vi "Get All Logging Properties.vi"(8 "error in":errorcluster, 11 "logging ref":T3=18446744073709551615 format="%.0x") -> (0 "error out":errorcluster, 1 "log thresholds":T2 {"Segment Files By" items=["Time", "Size"]}, 2 "log file info":T1, 3 "logging ref out":T3 format="%.0x")   [LabVIEW 2020, in "AIM ARINC 664 Scripting.lvlib"]
uses:
  AIM ARINC 664 Scripting.lvlib
  <vilib>/NI VeriStand/Custom Device API/Custom Device Item Ref.ctl
  Shared/loggingThreshold_types.ctl
  Shared/logFileInfo_types.ctl
  <vilib>/NI VeriStand/Custom Device API/Custom Device API.lvlib
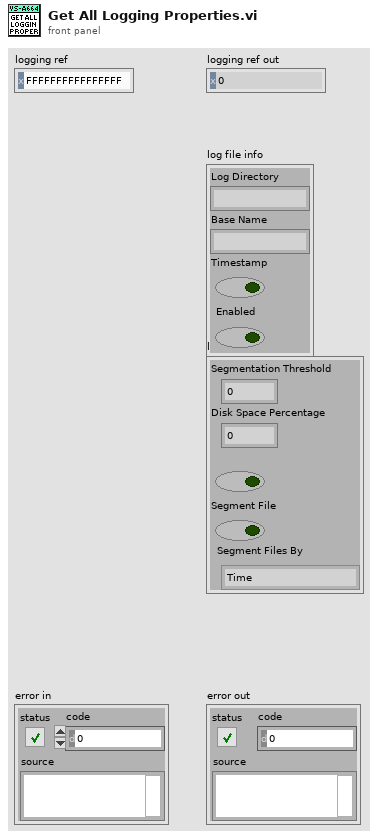
[diagram p1: front panel]
types:
  T1 = typedef "logFileInfo_types.ctl" = cluster{"Log Directory":string, "Base Name":string, "Timestamp":bool, "Enabled":bool}
  T2 = typedef "loggingThreshold_types.ctl" = cluster{"Segmentation Threshold":dbl, "Disk Space Percentage":dbl, "Check Disk Space":bool, "Segment File":bool, "Segment Files By":u16}
  T3 = typedef "Custom Device API.lvlib/Custom Device Item Ref.ctl" = u64
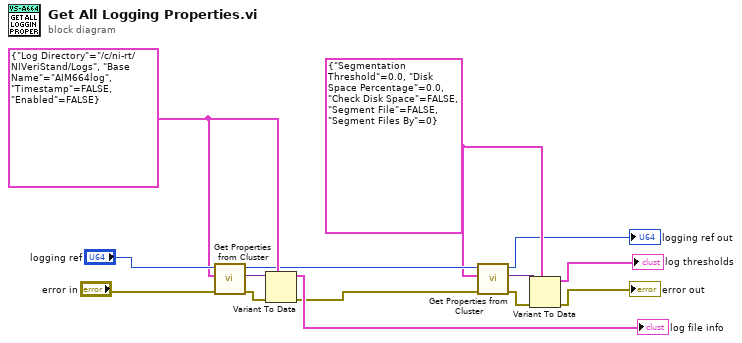
[diagram p0: block diagram]
diagram:
  w4 = T2 {"Segmentation Threshold"=0.0, "Disk Space Percentage"=0.0, "Check Disk Space"=FALSE, "Segment File"=FALSE, "Segment Files By"=0} ("log thresholds")
  w9 = T1 {"Log Directory"="/c/ni-rt/NIVeriStand/Logs", "Base Name"="AIM664log", "Timestamp"=FALSE, "Enabled"=FALSE} ("log file info")
  n1 = call "Get Properties from Cluster.vi"("error in"="error in", "Variant Cluster"=w9, "custom device ref in"="logging ref") -> ("error out"=w13:errorcluster, "data"=w14:variant, "custom device ref out"=w5:T3)  [unwired: 5 in, 1 out]
  n2 = Variant To Data(error in=w13, type=w9, Variant=w14) -> (data=→"log file info":T1, error out=w6:errorcluster)
  n3 = call "Get Properties from Cluster.vi"("error in"=w6, "Variant Cluster"=w4, "custom device ref in"=w5) -> ("error out"=w8:errorcluster, "data"=w7:variant, "custom device ref out"=→"logging ref out":T3)  [unwired: 5 in, 1 out]
  n4 = Variant To Data(error in=w8, type=w4, Variant=w7) -> (data=→"log thresholds":T2, error out=→"error out":errorcluster)
